vi "PM100D_Close.vi"(1 "Mode":T1=2 items=["Deassert REN", "Assert REN", "Go To Local; Deassert REN ", "Assert REN; Address Device", "Local Lockout (Addressed Devices)", "Local Lockout (This Device)", "Go To Local"], 2 "error in (no error)":errorcluster, 3 "VISA resource name":refnum<visa-resource-name>) -> ()   [LabVIEW 2012]
doc: "Closes the VISA session\nSets the connected instrument in local mode (default option)"
uses:
  <vilib>/Instr/_visa.llb/VISA GPIB Control REN Mode.ctl
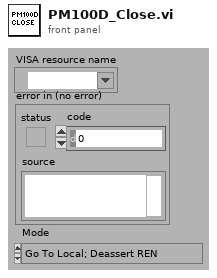
[diagram p1: front panel]
types:
  T1 = typedef "VISA GPIB Control REN Mode.ctl" = u16
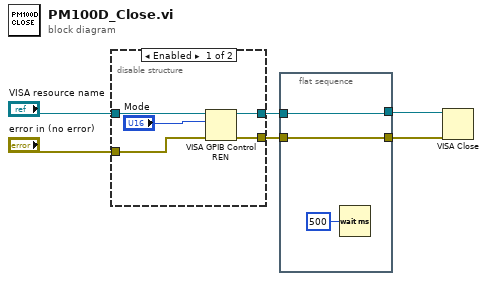
[diagram p0: block diagram]
diagram:
  n1 = disable-structure shown="Enabled" {
    disable-tunnel: "VISA resource name" -> [w10 _]
    disable-tunnel: "error in (no error)" -> [w9 _]
    disable-tunnel: [w8 _] -> w4
    disable-tunnel: [w7 _] -> w2
    frame Enabled {
      n2 = VISA GPIB Control REN(8:w9, 10:"Mode", 11:w10) -> (0:w7:errorcluster, 3:w8:refnum<visa-resource-name>)
    }
    frame Disabled {
    }
  }
  n3 = flat-sequence {
    tunnel: [w14] -> w3
    tunnel: w4 -> [w14]
    tunnel: w2 -> [w13]
    tunnel: [w13] -> w1
    frame #0 {
      n4 = Wait (ms)(milliseconds to wait=u32 500) -> ()  [unwired: 1 out]
    }
  }
  n5 = VISA Close(VISA resource name=w3, error in (no error)=w1) -> ()  [unwired: 1 out]
